vi "ToString.vi"(9 "Error in":errorcluster) -> (1 "Error as string":string)   [LabVIEW 2017, in "GPError.lvlib"]
doc: "Formats the <B>Error in</B> cluster into <B>Error as string</B> for easy logging or display of errors in a standardized format for instance. <B>Error as string</B> follows this pattern;\n\n\"<Error/Warning 1>; <Error/Warning 2>...<Error/Warning n>\"\n\nwhere each <Error/Warning m> is an appended error or warning of the following format:\n\n\"[<index>] Error/Warning code <code>, Source: <source>, Time: <timestamp>, <description 1>, <description 2>...<description n>\"\n\nwhere:\n\n<index> is the appended error index.\n<code> is the code field from the error.\n<source> is the decoded source value from the error (that's not the same as the source field from the error).\n<timestamp> is the embedded timestamp from the SetTimestamp function. This field will be omitted if there is no timestamp present.\n<description 1..n> are the calculated description strings from the concrete error.\n\nIf <B>Error in</B> is a single error or warning (no appended errors or warnings) then the entire <B>Error as string</B> will be just this format (i.e. without the \"[<index>]\" part):\n\n\"Error/Warning code <code>, Source: <source>, <description 1>, <description 2>...<description n>\"\n\nSteen Schmidt\nGPower\n15/11 2014"
uses:
  GPError.lvlib
panel:
  # "Copyright © 2014\nGPower\nSee enclosed license file for terms and conditions"
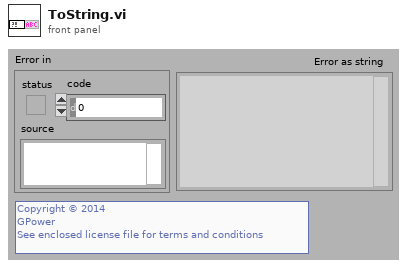
[diagram p1: front panel]
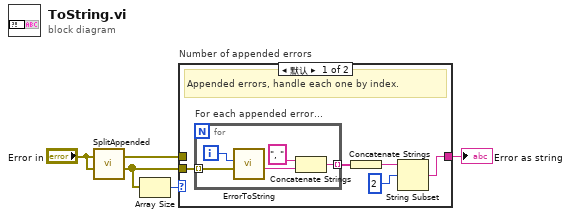
[diagram p0: block diagram]
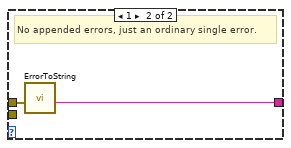
[diagram p2: hidden frame]
diagram:
  n1 = call "SplitAppended.vi"("Appended errors in"="Error in") -> ("Errors out"=w3:errorcluster[])  [unwired: 10 in]
  n2 = Array Size(array=w3) -> (size(s)=w4:i32)
  n3 = case "Number of appended errors" shown="默认" w4 {
    tunnel: w3 -> [w9 _]
    tunnel: "Error in" -> [_ w16]
    tunnel: [w5 w15] -> w1
    frame Default {
      # "Appended errors, handle each one by index."
      n4 = for "For each appended error..." {
        tunnel: w9 -> [w14] mode=indexing
        tunnel: [w10] -> w8 mode=indexing
        i -> [w13]
        n5 = call "ErrorToString.vi"("Error in"=w14, "Appended error index"=w13) -> ("Error as string"=w12:string)  [unwired: 9 in]
        n6 = Concatenate Strings(", " ("string"), w12) -> (w10:string)
      }
      n7 = Concatenate Strings(w8) -> (w7:string)
      n8 = String Subset(string=w7, offset (0)=2) -> (substring=w5:string)  [unwired: 1 in]
    }
    frame 1 {
      # "No appended errors, just an ordinary single error."
      n9 = call "ErrorToString.vi"("Error in"=w16) -> ("Error as string"=w15:string)  [unwired: 10 in]
    }
  }
  "Error as string" <- w1
